vi "Interface.vi"() -> ()   [LabVIEW 2019, in "Program Interface.lvclass"]
uses:
  Program Interface.lvclass
  Robot/Universal Robot/Universal Robot.lvclass
  C:/_Code/Development/Sub-Zero Functional Test/standard hardware/Universal Robots/UR LabVIEW Interface/Classes/Application/Application Interfaces/Application Interface/Application Interface.lvclass
  PlayQueueData.ctl
  Robot/Universal Robot/ProgramControlEvent.ctl
  Robot/Universal Robot/ProgramReturnStatus.ctl
  Program Interface.lvclass/Program Interface.ctl
  Program List From File/Program List From File.lvclass
  C:/_Code/Development/Sub-Zero Functional Test/standard hardware/Universal Robots/UR LabVIEW Interface/Classes/Application/Application Interfaces/Program Interface/Program List/Program List.lvclass
  Program List From SFTP/Program List From SFTP.lvclass
  Application Interface/FGVAction.ctl
  Application.lvclass
  Program List/Program List.lvclass
  Application Interface/Application Interface.lvclass
panel:
  in  "Program List":i32[](listbox)
  in  "Program Queue":i32(listbox)
  in  "play":bool
  in  "play queue":bool
  in  "clear queue":bool
  in  "save queue":bool
  in  "load queue":bool
  out "Loaded Program":string
  in  "pause":bool
  in  "stop":bool
  out "Program Status":string
  out "programStatusColor":u32(colorbox)
  in  "Saved Queues":i32[](listbox) caption="double click to delete"
  out "Complete":i32=1 min=1 max=100000 step=1
  in  "Cycles":i32=1 min=1 max=100000 step=1
  out "Header":string
  in  "sample rate (ms)":i32
  in  "interface":refnum<class "Program Interface.lvclass">
  in  "robot":refnum<class "Universal Robot.lvclass">
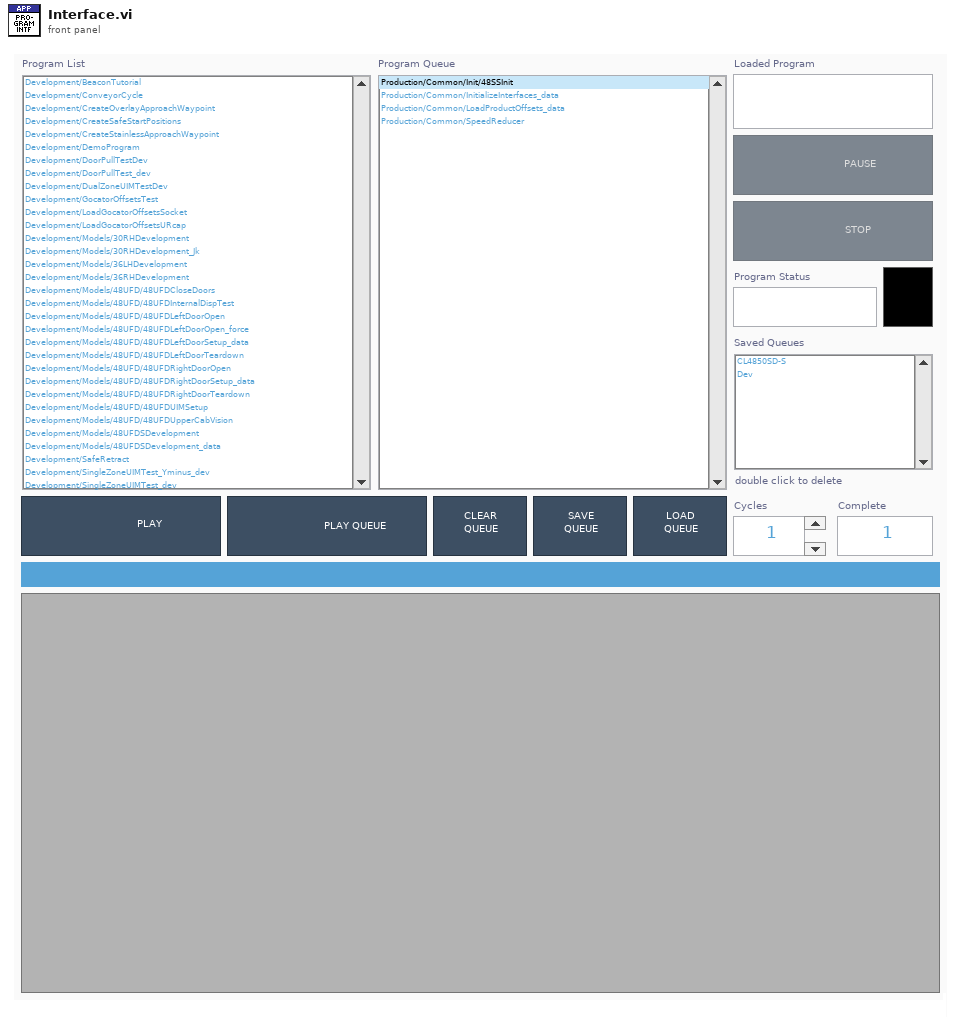
[diagram p1: front panel]
types:
  T1 = typedef "Program Interface.lvclass/PlayQueueData.ctl" = cluster{"Program Interface":refnum<class "Program Interface.lvclass">, "Universal Robot":refnum<class "Universal Robot.lvclass">, "Play Single":bool}
  T2 = typedef "Application.lvclass/ApplicationSettings.ctl" = cluster{"Robot IP":string, "Socket Host IP":string, "Robot Type":T3, "Use SFTP Program List":bool, "Robot Logging":bool, "TCP Logging":bool}
  T3 = typedef "Application.lvclass/RobotType.ctl" = enum16{"UR E-Series", "UR CB-Series"}
  T4 = typedef "Universal Robot.lvclass/ProgramControlEvent.ctl" = enum16{"Stop", "Pause", "Resume"}
  T5 = typedef "Application Interface.lvclass/FGVAction.ctl" = enum16{"Initialize", "Get Last Status", "Update Status"}
  T6 = typedef "Application.lvclass/FrontPanelControls.ctl" = cluster{"Operation Interface":refnum<vi>, "Program Interface":refnum<vi>, "Command Interface":refnum<vi>, "Socket Interface":refnum<vi>, "Error Interface":refnum<vi>}
  T7 = typedef "Universal Robot.lvclass/ProgramStatus.ctl" = cluster{"Loaded Program":string, "Valid Program":bool, "Program State":T8, "Running":bool}
  T8 = typedef "Universal Robot.lvclass/ProgramState.ctl" = enum16{"STOPPED", "PLAYING", "PAUSE"}
  T9 = typedef "Universal Robot.lvclass/RobotStatus.ctl" = cluster{"Robot Mode":T10, "Operational Mode":T11, "Safety Status":T12, "Remote Control":bool}
  T10 = typedef "Universal Robot.lvclass/RobotMode.ctl" = enum16{"INVALID", "NO_CONTROLLER", "DISCONNECTED", "CONFIRM_SAFETY", "BOOTING", "POWER_OFF", "POWER_ON", "IDLE", "BACKDRIVE", "RUNNING"}
  T11 = typedef "Universal Robot.lvclass/OperationalMode.ctl" = enum16{"NONE", "MANUAL", "AUTOMATIC"}
  T12 = typedef "Universal Robot.lvclass/SafetyStatus.ctl" = enum16{"INVALID", "NORMAL", "REDUCED", "PROTECTIVE_STOP", "RECOVERY", "SAFEGUARD_STOP", "SYSTEM_EMERGENCY_STOP", "ROBOT_EMERGENCY_STOP", "VIOLATION", "FAULT", "AUTOMATIC_MODE_SAFEGAURD_STOP", "SYSTEM_THREE_POSITION_ENABLING_STOP"}
  T13 = typedef "Universal Robot.lvclass/ProgramReturnStatus.ctl" = enum16{"Incomplete", "Complete", "Stopped", "Error", "Faulted", "Timeout"}
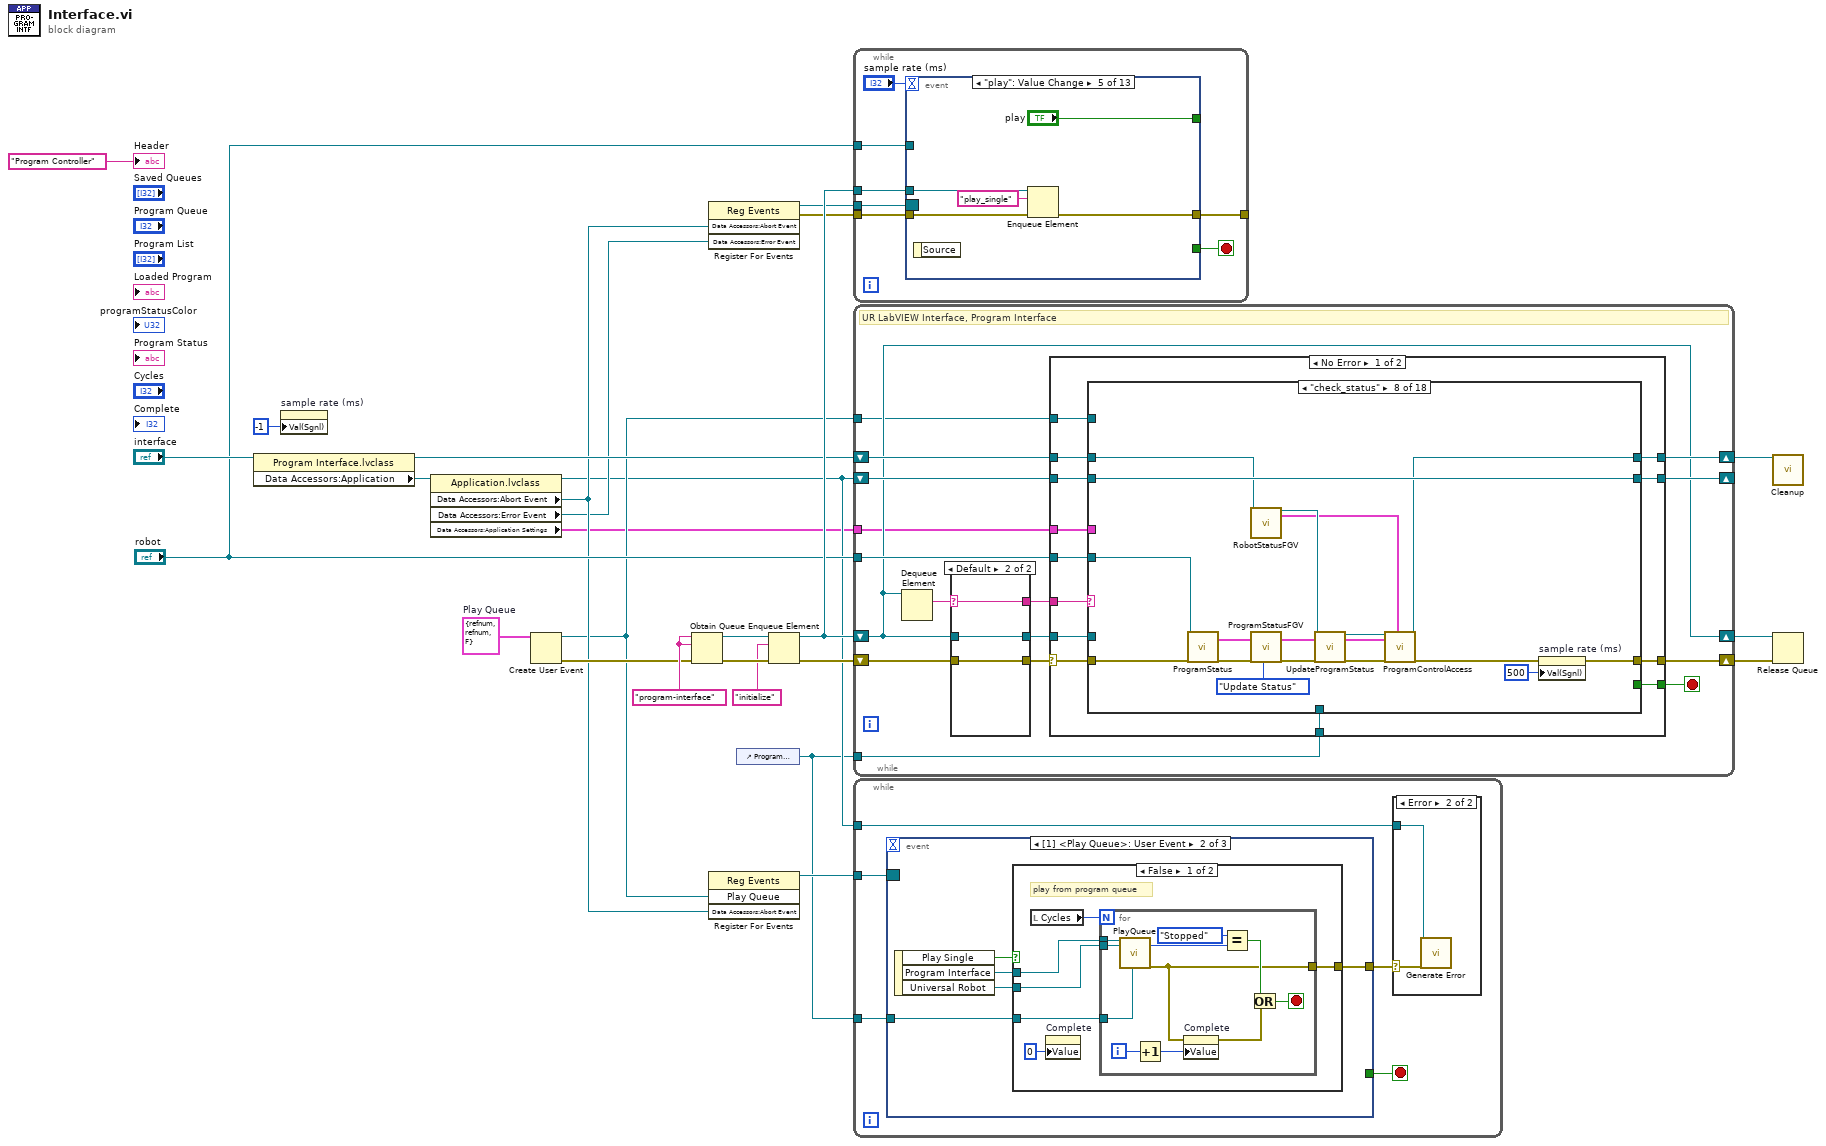
[diagram p0: block diagram]
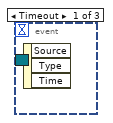
[diagram p3: hidden frame]
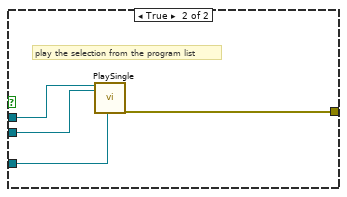
[diagram p4: hidden frame]
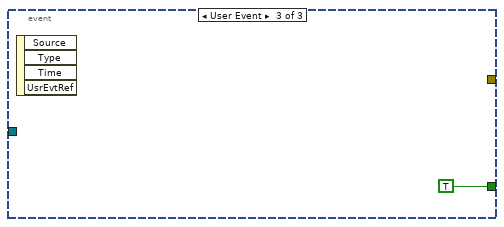
[diagram p5: hidden frame]
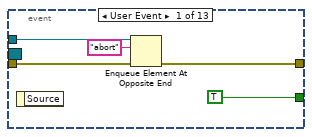
[diagram p6: hidden frame]
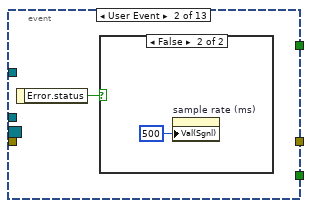
[diagram p7: hidden frame]
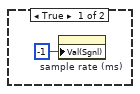
[diagram p8: hidden frame]
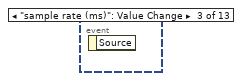
[diagram p9: hidden frame]
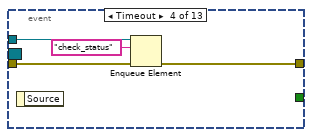
[diagram p10: hidden frame]
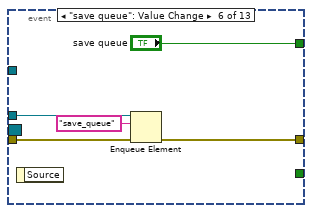
[diagram p11: hidden frame]
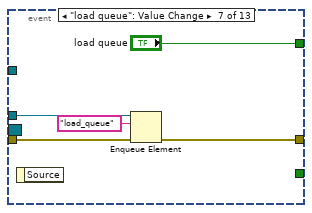
[diagram p12: hidden frame]
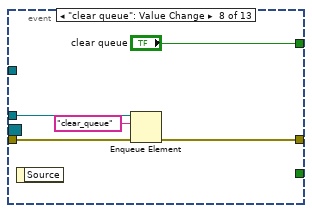
[diagram p13: hidden frame]
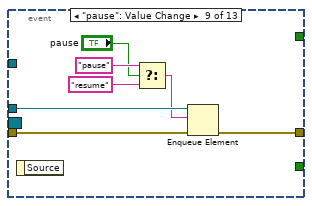
[diagram p14: hidden frame]
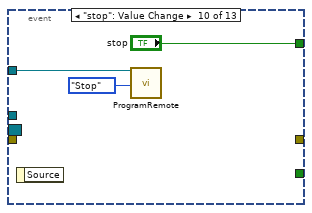
[diagram p15: hidden frame]
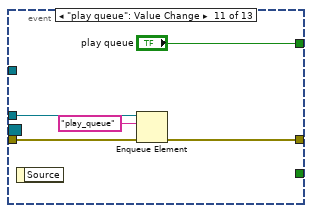
[diagram p16: hidden frame]
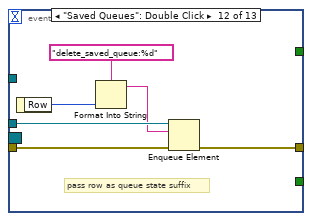
[diagram p17: hidden frame]
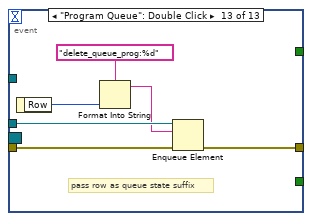
[diagram p18: hidden frame]
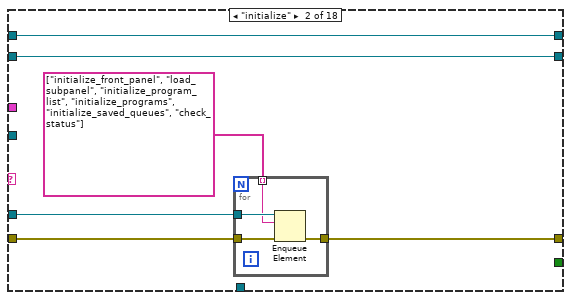
[diagram p20: hidden frame]
diagram:
  w9 = T1 {"Program Interface"=refnum, "Universal Robot"=refnum, "Play Single"=FALSE}  # Play Queue
  w21 = "program-interface" ("name (unnamed)")
  n1 = property class="Program Interface.lvclass"(reference="interface") -> (reference out=w15:refnum<class "Program Interface.lvclass">, "Data Accessors:Application"=w16:refnum<class "Application.lvclass">)  [unwired: 1 in, 1 out]
  n2 = property on="sample rate (ms)" class="DigNum (strict)"("Val(Sgnl)"=-1 ("Value (Signaling)")) -> ()  [unwired: 2 in, 2 out]
  n3 = property class="Application.lvclass"(reference=w16) -> (reference out=w4:refnum<class "Application.lvclass">, "Data Accessors:Abort Event"=w8:refnum<user-event>, "Data Accessors:Error Event"=w5:refnum<user-event>, "Data Accessors:Application Settings"=w2:T2)  [unwired: 1 in, 1 out]
  n4 = Create User Event(user event datatype=w9) -> (user event=w7:refnum<user-event>, error out=w10:errorcluster)  [unwired: 1 in]
  n5 = Obtain Queue(name (unnamed)=w21, element data type=w21, error in (no error)=w10) -> (queue out=w25:refnum<queue>, error out=w26:errorcluster)  [unwired: 2 in, 1 out]
  n6 = register-events(w8, w5) -> (reference out=w17:refnum<event-registration>, error out=w18:errorcluster)  [unwired: 2 in]
  n7 = register-events(w7, w8) -> (reference out=w6:refnum<event-registration>)  [unwired: 2 in, 1 out]
  n8 = control-ref of="Program Controller"() -> (w3:refnum<vi>)
  n9 = Enqueue Element(queue=w25, element="initialize", error in (no error)=w26) -> (queue out=w22:refnum<queue>, error out=w23:errorcluster)  [unwired: 1 in, 1 out]
  n10 = while {
    tunnel: w22 -> [w33]
    tunnel: w18 -> [w32]
    tunnel: w17 -> [w31]
    tunnel: [w30] -> _
    tunnel: "robot" -> [w28]
    stop <- w29 stop-if-true
    n11 = event shown="[4] \"play\": Value Change" {
      selector: w31 -> [_ _ _ _ _ _ _ _ _ _ _ _ _]
      dyn-events: _ -> [_ _ _ _ _ _ _ _ _ _ _ _ _]
      timeout: "sample rate (ms)" -> [_ _ _ _ _ _ _ _ _ _ _ _ _]
      tunnel: w33 -> [w38 _ _ w45 w50 w55 w60 w65 w72 _ w80 w86 w92]
      tunnel: w32 -> [w37 _ _ w44 w49 w54 w59 w64 w71 _ w79 w85 w91]
      tunnel: [w36 _ _ w43 w48 w53 w58 w63 w70 _ w78 w84 w90] -> w30
      tunnel: [TRUE _ _ _ _ _ _ _ _ _ _ _ _] -> w29
      tunnel: [_ _ _ _ "play" "save queue" "load queue" "clear queue" _ "stop" "play queue" _ _] -> _
      tunnel: w28 -> [_ _ _ _ _ _ _ _ _ w74 _ _ _]
      event User Event {
        n12 = event-data() -> ()  [unwired: 1 in, 1 out]
        n13 = Enqueue Element At Opposite End(queue=w38, element="abort", error in (no error)=w37) -> (error out=w36:errorcluster)  [unwired: 1 in, 2 out]
      }
      event User Event {
        n14 = event-data() -> ("Error.status"=w39:bool)  [unwired: 1 in]
        n15 = case shown="False" w39 {
          frame True {
            n16 = property on="sample rate (ms)" class="DigNum (strict)"("Val(Sgnl)"=-1 ("Value (Signaling)")) -> ()  [unwired: 2 in, 2 out]
          }
          frame False {
            n17 = property on="sample rate (ms)" class="DigNum (strict)"("Val(Sgnl)"=500 ("Value (Signaling)")) -> ()  [unwired: 2 in, 2 out]
          }
        }
      }
      event "sample rate (ms)": Value Change {
        n18 = event-data() -> ()  [unwired: 1 in, 1 out]
      }
      event Timeout {
        n19 = event-data() -> ()  [unwired: 1 in, 1 out]
        n20 = Enqueue Element(queue=w45, element="check_status", error in (no error)=w44) -> (error out=w43:errorcluster)  [unwired: 1 in, 2 out]
      }
      event "play": Value Change {
        n21 = event-data() -> ()  [unwired: 1 in, 1 out]
        n22 = Enqueue Element(queue=w50, element="play_single", error in (no error)=w49) -> (error out=w48:errorcluster)  [unwired: 1 in, 2 out]
      }
      event "save queue": Value Change {
        n23 = event-data() -> ()  [unwired: 1 in, 1 out]
        n24 = Enqueue Element(queue=w55, element="save_queue", error in (no error)=w54) -> (error out=w53:errorcluster)  [unwired: 1 in, 2 out]
      }
      event "load queue": Value Change {
        n25 = event-data() -> ()  [unwired: 1 in, 1 out]
        n26 = Enqueue Element(queue=w60, element="load_queue", error in (no error)=w59) -> (error out=w58:errorcluster)  [unwired: 1 in, 2 out]
      }
      event "clear queue": Value Change {
        n27 = event-data() -> ()  [unwired: 1 in, 1 out]
        n28 = Enqueue Element(queue=w65, element="clear_queue", error in (no error)=w64) -> (error out=w63:errorcluster)  [unwired: 1 in, 2 out]
      }
      event "pause": Value Change {
        n29 = event-data() -> ()  [unwired: 1 in, 1 out]
        n30 = Select(t="pause" ("element"), s="pause", f="resume" ("element")) -> (s? t:f=w68:string)
        n31 = Enqueue Element(queue=w72, element=w68, error in (no error)=w71) -> (error out=w70:errorcluster)  [unwired: 1 in, 2 out]
      }
      event "stop": Value Change {
        n32 = event-data() -> ()  [unwired: 1 in, 1 out]
        n33 = call-dynamic "ProgramRemote.vi"("Universal Robot.lvclass in"=w74, "Remote"=ProgramControlEvent."Stop") -> ()  [unwired: 16 in, 2 out]
      }
      event "play queue": Value Change {
        n34 = event-data() -> ()  [unwired: 1 in, 1 out]
        n35 = Enqueue Element(queue=w80, element="play_queue", error in (no error)=w79) -> (error out=w78:errorcluster)  [unwired: 1 in, 2 out]
      }
      event "Saved Queues": Double Click {
        # "pass row as queue state suffix"
        n36 = event-data() -> ("Row"=w83:i32)  [unwired: 1 in]
        n37 = Format Into String(format string="delete_saved_queue:%d" ("element"), w83) -> (resulting string=w81:string)  [unwired: 2 in, 1 out]
        n38 = Enqueue Element(queue=w86, element=w81, error in (no error)=w85) -> (error out=w84:errorcluster)  [unwired: 1 in, 2 out]
      }
      event "Program Queue": Double Click {
        # "pass row as queue state suffix"
        n39 = event-data() -> ("Row"=w89:i32)  [unwired: 1 in]
        n40 = Format Into String(format string="delete_queue_prog:%d" ("element"), w89) -> (resulting string=w87:string)  [unwired: 2 in, 1 out]
        n41 = Enqueue Element(queue=w92, element=w87, error in (no error)=w91) -> (error out=w90:errorcluster)  [unwired: 1 in, 2 out]
      }
    }
  }
  n42 = while {
    shift-right: [w108] -> w19
    shift-left: w23 -> [w97]
    shift-right: [w99] -> w20
    shift-left: w22 -> [w99]
    tunnel: "robot" -> [w105]
    shift-right: [w104] -> _
    shift-left: w4 -> [w106]
    shift-right: [w102] -> w13
    shift-left: w15 -> [w103]
    tunnel: w7 -> [w95]
    tunnel: w3 -> [w94]
    tunnel: w2 -> [w93]
    stop <- w107 stop-if-true
    # "UR LabVIEW Interface, Program Interface"
    n43 = Dequeue Element(queue=w99) -> (element=w101:string)  [unwired: 2 in, 3 out]
    n44 = case shown="Default" w101 {
      selector: w101 -> [w273 w276]
      tunnel: [w273 w276] -> w100
      tunnel: w99 -> [w272 w275]
      tunnel: [w272 w275] -> w98
      tunnel: w97 -> [_ w274]
      tunnel: [_ w274] -> w96
      frame "abort" {
        # "clear error"
      }
      frame Default {
      }
    }
    n45 = case shown="No Error" w96 {
      selector: w96 -> [w112 w270]
      tunnel: [w121 _] -> w108
      tunnel: [w120 _] -> w107
      tunnel: w106 -> [w119 w269]
      tunnel: w105 -> [w118 _]
      tunnel: [w117 w269] -> w104
      tunnel: w103 -> [w116 w271]
      tunnel: [w115 w271] -> w102
      tunnel: w100 -> [w114 _]
      tunnel: w98 -> [w113 _]
      tunnel: w95 -> [w111 _]
      tunnel: w94 -> [w110 _]
      tunnel: w93 -> [w109 _]
      frame No Error {
        n46 = case shown="\"check_status\"" w114 {
          selector: w114 -> [_ _ _ _ _ _ _ _ _ _ _ _ _ w230 w240 _ _ _]
          tunnel: w112 -> [w124 w126 _ w159 _ w174 w181 w198 w203 _ w212 w215 w222 _ _ _ _ w267]
          tunnel: w113 -> [_ w127 _ _ _ _ _ _ _ _ _ _ _ _ _ _ _ _]
          tunnel: [w124 w125 _ w162 w168 w173 w180 w188 w202 w206 w211 w214 w221 w225 _ w246 w254 w266] -> w121
          tunnel: [_ _ _ _ _ _ _ _ _ _ _ _ _ _ _ _ _ TRUE] -> w120
          tunnel: w119 -> [w123 w130 w148 w158 w165 w177 w182 w200 w205 w209 w213 w218 w223 w231 w241 w252 w260 w263]
          tunnel: w118 -> [_ _ _ _ _ _ _ w197 w201 w207 _ _ _ _ _ w248 w256 _]
          tunnel: [w123 w130 w148 w157 w165 w177 w182 w200 w205 w209 w213 w218 w223 w231 w241 w252 w260 w262] -> w117
          tunnel: w116 -> [w122 w129 w154 w160 w172 w176 w179 w196 w204 w208 w210 w217 w220 w227 w237 w247 w255 w265]
          tunnel: [w122 w129 w143 w160 w171 w175 w178 w199 w204 w208 w210 w216 w219 w226 w237 w247 w255 w265] -> w115
          tunnel: w111 -> [_ _ _ _ _ _ _ _ _ _ _ _ _ _ _ w249 w257 _]
          tunnel: w110 -> [_ _ _ _ _ _ _ _ _ _ _ _ _ _ _ _ _ _]
          tunnel: w109 -> [_ _ _ _ w167 _ _ _ _ _ _ _ _ _ _ _ _ _]
          frame Default {
          }
          frame "initialize" {
            n47 = for {
              tunnel: w127 -> [w134]
              tunnel: w126 -> [w133]
              tunnel: [w132] -> w125
              tunnel: string[] ["initialize_front_panel", "load_subpanel", "initialize_program_list", "initialize_programs", "initialize_saved_queues", "check_status"] -> [w131] mode=indexing
              n48 = Enqueue Element(queue=w134, element=w131, error in (no error)=w133) -> (error out=w132:errorcluster)  [unwired: 1 in, 2 out]
            }
          }
          frame "initialize_front_panel" {
            n49 = control-ref of="This VI"() -> (w153:refnum<vi>)
            n50 = control-ref of="programStatusColor"() -> (w147:refnum<vi>)
            n51 = control-ref of="play"() -> (w151:refnum<vi>)
            n52 = control-ref of="pause"() -> (w135:refnum<vi>)
            n53 = control-ref of="stop"() -> (w150:refnum<vi>)
            n54 = control-ref of="play queue"() -> (w142:refnum<vi>)
            n55 = control-ref of="clear queue"() -> (w137:refnum<vi>)
            n56 = control-ref of="save queue"() -> (w136:refnum<vi>)
            n57 = control-ref of="Program List"() -> (w141:refnum<vi>)
            n58 = control-ref of="Program Queue"() -> (w145:refnum<vi>)
            n59 = control-ref of="Saved Queues"() -> (w138:refnum<vi>)
            n60 = property class="VI"(reference=w153) -> ("Panel"=w152:refnum<vi>)  [unwired: 1 in, 2 out]
            n61 = control-ref of="Loaded Program"() -> (w149:refnum<vi>)
            n62 = control-ref of="Program Status"() -> (w146:refnum<vi>)
            n63 = Bundle By Name(cluster=w154, "Front Panel"=w152, "Play"=w151, "Pause"=w135, "Stop"=w150, "Loaded Program"=w149, "Program List"=w141, "Program Status Color"=w147, "Program Status"=w146, "Program Queue"=w145, "Play Queue"=w142, "Saved Queues"=w138, "Clear Queue"=w137, "Save Queue"=w136) -> (w144:refnum<class "Program Interface.lvclass">)
            n64 = call "Initialize.vi"("Operation Interface in"=w144) -> ("Operation Interface out"=w143:refnum<class "Program Interface.lvclass">)  [unwired: 18 in]
            n65 = local write "Cycles"(1 ("Cycles")) -> ()
            n66 = local write "Complete"(0 ("Complete")) -> ()
          }
          frame "load_subpanel" {
            n67 = property class="Application.lvclass"(reference=w158) -> (reference out=w157:refnum<class "Application.lvclass">, "Data Accessors:Subpanels"=w156:T6)  [unwired: 1 in, 1 out]
            n68 = Unbundle By Name(w156) -> ("Program Interface"=w155:refnum<vi>)
            n69 = control-ref of="This VI"() -> (w161:refnum<vi>)
            n70 = invoke class="SubPnl" method="Insert VI"(reference=w155, error in=w159, "VI Ref"=w161) -> (error out=w162:errorcluster)  [unwired: 1 in, 3 out]
          }
          frame "initialize_program_list" {
            n71 = Unbundle By Name(w167) -> ("Use SFTP Program List"=w170:bool)
            n72 = Select(t=refnum<class "Program List From SFTP.lvclass"> refnum ("Program List From SFTP"), s=w170, f=refnum<class "Program List From File.lvclass"> refnum ("Program List From File")) -> (s? t:f=w163:refnum<class "Program List.lvclass">)
            n73 = call-dynamic "Initialize.vi"("Program List in"=w163, "Application.lvclass"=w165) -> ("Program List out"=w169:refnum<class "Program List.lvclass">, "error out"=w168:errorcluster)  [unwired: 16 in]
            n74 = property class="Program Interface.lvclass"(reference=w172, "Data Accessors:Program List"=w169) -> (reference out=w171:refnum<class "Program Interface.lvclass">)  [unwired: 1 in, 1 out]
          }
          frame "initialize_programs" {
            n75 = call "LoadPrograms.vi"("Program Interface in"=w176, "error in (no error)"=w174) -> ("Program Interface out"=w175:refnum<class "Program Interface.lvclass">, "error out"=w173:errorcluster)  [unwired: 16 in]
          }
          frame "initialize_saved_queues" {
            n76 = call "LoadSavedQueueList.vi"("Program Interface in"=w179, "error in (no error)"=w181) -> ("Program Interface out"=w178:refnum<class "Program Interface.lvclass">, "error out"=w180:errorcluster)  [unwired: 16 in]
          }
          frame "check_status" {
            n77 = call-dynamic "ProgramStatus.vi"("Universal Robot.lvclass in"=w197, "error in (no error)"=w198) -> ("Program Status"=w187:T7, "error out"=w185:errorcluster)  [unwired: 15 in, 1 out]
            n78 = call "RobotStatusFGV.vi"("Application Interface in"=w196) -> ("Application Interface out"=w195:refnum<class "Program Interface.lvclass">, "Robot Status out"=w192:T9)  [unwired: 16 in, 1 out]
            n79 = call "ProgramStatusFGV.vi"("Program Status"=w187, "error in (no error)"=w185, "Action (Read)"=FGVAction."Update Status") -> ("Program Status out"=w186:T7, "error out"=w184:errorcluster)  [unwired: 14 in, 1 out]
            n80 = call "UpdateProgramStatus.vi"("Program Interface in"=w195, "Program Status in"=w186, "error in (no error)"=w184) -> ("Program Interface out"=w194:refnum<class "Program Interface.lvclass">, "Program Status out"=w191:T7, "error out"=w193:errorcluster)  [unwired: 14 in]
            n81 = call "ProgramControlAccess.vi"("Program Interface in"=w194, "Program Status"=w191, "error in (no error)"=w193, "Robot Status"=w192) -> ("Program Interface out"=w199:refnum<class "Program Interface.lvclass">, "error out"=w190:errorcluster)  [unwired: 14 in]
            n82 = property on="sample rate (ms)" class="DigNum (strict)"(error in=w190, "Val(Sgnl)"=500 ("Value (Signaling)")) -> (error out=w188:errorcluster)  [unwired: 1 in, 1 out]
          }
          frame "pause" {
            n83 = call-dynamic "Pause.vi"("Universal Robot.lvclass in"=w201, "error in (no error)"=w203) -> ("error out"=w202:errorcluster)  [unwired: 16 in, 1 out]
          }
          frame "resume" {
            n84 = call-dynamic "Play.vi"("Universal Robot.lvclass in"=w207) -> ("error out"=w206:errorcluster)  [unwired: 17 in, 1 out]
          }
          frame "clear_queue" {
            n85 = call "ClearQueue.vi"("Program Interface in"=w210, "error in (no error)"=w212) -> ("error out"=w211:errorcluster)  [unwired: 16 in, 1 out]
          }
          frame "load_queue" {
            n86 = call "LoadSavedQueue.vi"("Program Interface in"=w217, "error in (no error)"=w215) -> ("Program Interface out"=w216:refnum<class "Program Interface.lvclass">, "error out"=w214:errorcluster)  [unwired: 16 in]
          }
          frame "save_queue" {
            n87 = call "SaveQueue.vi"("Program Interface in"=w220, "error in (no error)"=w222) -> ("Program Interface out"=w219:refnum<class "Program Interface.lvclass">, "error out"=w221:errorcluster)  [unwired: 16 in]
          }
          frame "delete_saved_queue ".."delete_saved_queue~" {
            n88 = Match Pattern(string=w230, regular expression=":") -> (after substring=w228:string)  [unwired: 1 in, 3 out]
            n89 = Decimal String To Number(string=w228) -> (number=w224:i32)  [unwired: 2 in, 1 out]
            n90 = call "DeleteQueue.vi"("Program Interface in"=w227, "Queue Index"=w224) -> ("Program Interface out"=w226:refnum<class "Program Interface.lvclass">, "error out"=w225:errorcluster)  [unwired: 16 in]
          }
          frame "delete_queue_prog ".."delete_queue_prog~" {
            n91 = Unbundle By Name(w237) -> ("Program Queue"=w236:refnum<vi>)
            n92 = Match Pattern(string=w240, regular expression=":") -> (after substring=w238:string)  [unwired: 1 in, 3 out]
            n93 = Decimal String To Number(string=w238) -> (number=w232:i32)  [unwired: 2 in, 1 out]
            n94 = property class="LstBox (strict)"(reference=w236) -> (reference out=w235:refnum<vi>, "Item Names"=w233:string[])  [unwired: 1 in, 1 out]
            n95 = Index Array(array=w233, index=w232) -> (element=w234:string)
            n96 = case shown="Default" w234 {
              tunnel: w235 -> [w243 _]
              tunnel: w233 -> [w245 _]
              tunnel: w232 -> [w244 _]
              frame Default {
                n97 = Delete From Array(array=w245, index=w244) -> (array with subset deleted=w242:string[])  [unwired: 1 in, 1 out]
                n98 = property class="LstBox (strict)"(reference=w243, "Item Names"=w242) -> ()  [unwired: 1 in, 2 out]
              }
              frame "" {
              }
            }
          }
          frame "play_queue" {
            w251 = T1 {"Program Interface"=refnum, "Universal Robot"=refnum, "Play Single"=FALSE}  # Play Queue
            n99 = Bundle By Name(cluster=w251, "Program Interface"=w247, "Universal Robot"=w248) -> (w250:T1)
            n100 = Generate User Event(user event=w249, event data cluster=w250) -> (error out=w246:errorcluster)  [unwired: 2 in, 1 out]
          }
          frame "play_single" {
            w259 = T1 {"Program Interface"=refnum, "Universal Robot"=refnum, "Play Single"=FALSE}  # Play Queue
            n101 = Bundle By Name(cluster=w259, "Program Interface"=w255, "Universal Robot"=w256, "Play Single"=TRUE) -> (w258:T1)
            n102 = Generate User Event(user event=w257, event data cluster=w258) -> (error out=w254:errorcluster)  [unwired: 2 in, 1 out]
          }
          frame "abort" {
            n103 = property class="Application.lvclass"(reference=w263) -> (reference out=w262:refnum<class "Application.lvclass">, "Data Accessors:Subpanels"=w264:T6)  [unwired: 1 in, 1 out]
            n104 = Unbundle By Name(w264) -> ("Program Interface"=w261:refnum<vi>)
            n105 = invoke class="SubPnl" method="Remove VI"(reference=w261, error in=w267) -> (error out=w266:errorcluster)  [unwired: 1 in, 2 out]
          }
        }
      }
      frame Error {
        n106 = call "Generate Error.vi"("Application in"=w269, "error in (no error)"=w270) -> ()  [unwired: 17 in, 1 out]
      }
    }
  }
  n107 = while {
    tunnel: w6 -> [w281]
    tunnel: w4 -> [w278]
    tunnel: w3 -> [w277]
    stop <- w280 stop-if-true
    n108 = event shown="[1] <Play Queue>: User Event" {
      selector: w281 -> [_ _ _]
      dyn-events: _ -> [_ _ _]
      timeout: _ -> [_ _ _]
      tunnel: [_ w286 _] -> w279
      tunnel: [_ _ TRUE] -> w280
      tunnel: w277 -> [_ w285 _]
      event Timeout {
        n109 = event-data() -> ()  [unwired: 1 in, 3 out]
      }
      event User Event {
        n110 = event-data() -> ("Play Single"=w284:bool, "Program Interface"=w288:refnum<class "Program Interface.lvclass">, "Universal Robot"=w287:refnum<class "Universal Robot.lvclass">)  [unwired: 1 in]
        n111 = case shown="False" w284 {
          tunnel: w288 -> [w294 w309]
          tunnel: w287 -> [w293 w308]
          tunnel: [w292 w307] -> w286
          tunnel: w285 -> [w290 w306]
          frame False {
            # "play from program queue"
            n112 = local read "Cycles"() -> (w291:i32)
            n113 = property on="Complete" class="DigNum (strict)"("Value"=0 ("Complete")) -> ()  [unwired: 2 in, 2 out]
            n114 = for {
              N: w291 -> [_]
              tunnel: w294 -> [w305]
              tunnel: w293 -> [w304]
              tunnel: [w296] -> w292
              tunnel: w290 -> [w297]
              i -> [w299]
              stop <- w300 stop-if-true
              n115 = call "PlayQueue.vi"("Program Interface in"=w305, "robot"=w304, "Subpanel"=w297) -> ("programReturnStatus"=w303:T13, "error out"=w296:errorcluster)  [unwired: 14 in, 1 out]
              n116 = Increment(x=w299) -> (x+1=w298:i32)
              n117 = property on="Complete" class="DigNum (strict)"(error in=w296, "Value"=w298) -> (error out=w295:errorcluster)  [unwired: 1 in, 1 out]
              n118 = Equal?(x=ProgramReturnStatus."Stopped", y=w303) -> (x = y?=w301:bool)
              n119 = Or(x=w301, y=w295) -> (x .or. y?=w300:bool)
            }
          }
          frame True {
            # "play the selection from the program list"
            n120 = call "PlaySingle.vi"("Program Interface in"=w309, "robot"=w308, "Subpanel"=w306) -> ("error out"=w307:errorcluster)  [unwired: 14 in, 2 out]
          }
        }
      }
      event User Event {
        n121 = event-data() -> ()  [unwired: 1 in, 4 out]
      }
    }
    n122 = case shown="Error" w279 {
      selector: w279 -> [_ w283]
      tunnel: w278 -> [_ w282]
      frame No Error {
      }
      frame Error {
        n123 = call "Generate Error.vi"("Application in"=w282, "error in (no error)"=w283) -> ()  [unwired: 17 in, 1 out]
      }
    }
  }
  n124 = call "Cleanup.vi"("Operation Interface in"=w13) -> ()  [unwired: 19 in]
  n125 = Release Queue(queue=w20, error in (no error)=w19) -> ()  [unwired: 1 in, 3 out]
  "Header" <- "Program Controller" ("Header")
